vi "Get Named Range Values (Boolean).vi"(8 "error in":errorcluster, 9 "Sheet Name":string, 10 "Named Range Identifier":string, 11 "SpreadsheetDoc in":refnum<k24>) -> (0 "error out":errorcluster, 2 "Cells":bool[][](array[boolean]), 3 "SpreadsheetDoc out":refnum<k24>)   [LabVIEW 2019, in "Open Xml.lvlib"]
uses:
  Open Xml.lvlib
  D:/git/Open-Xml-LabVIEW/Source/DocumentFormat.OpenXml.dll
  DocumentFormat.OpenXml.dll
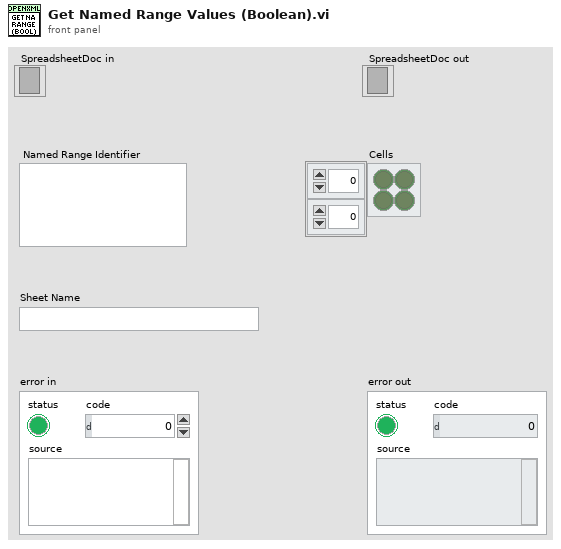
[diagram p1: front panel]
types:
  T1 = typedef "Open Xml.lvlib/Cell DataType.ctl" = enum16{"Void", "Boolean", "Number", "Error", "SharedString", "String", "InlineString", "Date"}
  T2 = cluster{"Number":dbl, "String":string, "Boolean":bool, "Time Stamp":timestamp, "Error":errorcluster}[][]
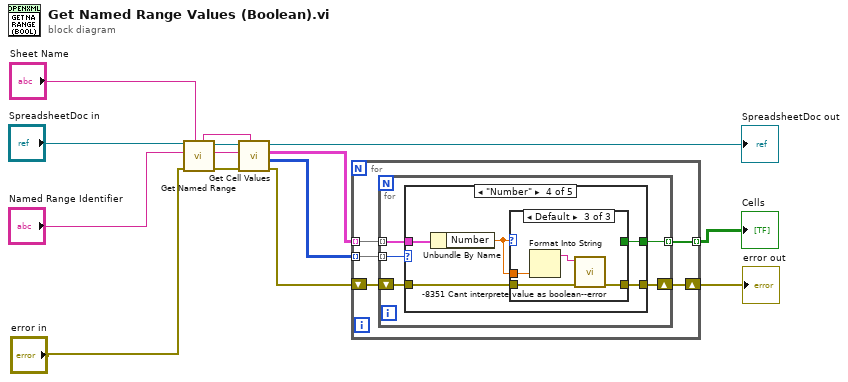
[diagram p0: block diagram]
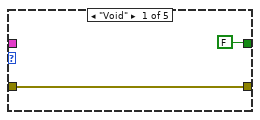
[diagram p2: hidden frame]
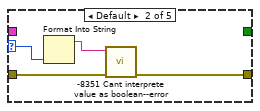
[diagram p3: hidden frame]
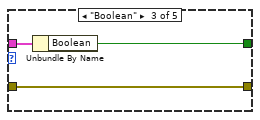
[diagram p4: hidden frame]
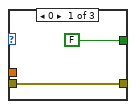
[diagram p5: hidden frame]
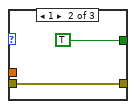
[diagram p6: hidden frame]
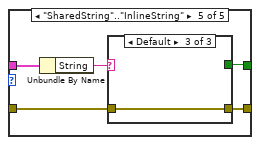
[diagram p7: hidden frame]
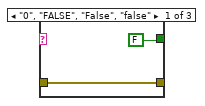
[diagram p8: hidden frame]
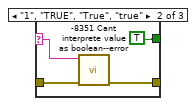
[diagram p9: hidden frame]
diagram:
  n1 = call "Get Named Range.vi"("Sheet Name"="Sheet Name", "error in"="error in", "Range Identifier"="Named Range Identifier", "SpreadsheetDoc in"="SpreadsheetDoc in") -> ("error out"=w11:errorcluster, "Range"=w8:string, "SpreadsheetDoc out"=w10:refnum<k24>, "Sheet Name"=w9:string)  [unwired: 4 in]
  n2 = call "Get Cell Values.vi"("Sheet Name"=w9, "error in"=w11, "Cell Addresses"=w8, "SpreadsheetDoc in"=w10) -> ("error out"=w3:errorcluster, "Types"=w5:T1[][], "Cell Values"=w7:T2, "SpreadsheetDoc out"=→"SpreadsheetDoc out":refnum<k24>)  [unwired: 4 in]
  n3 = for {
    tunnel: w7 -> [w19] mode=indexing
    tunnel: w5 -> [w18] mode=indexing
    tunnel: [w17] -> w1 mode=indexing
    shift-right: [w15] -> w2
    shift-left: w3 -> [w16]
    n4 = for {
      tunnel: w19 -> [w23] mode=indexing
      tunnel: w18 -> [w24] mode=indexing
      tunnel: [w20] -> w17 mode=indexing
      shift-right: [w21] -> w15
      shift-left: w16 -> [w22]
      n5 = case shown="\"Number\"" w24 {
        selector: w24 -> [_ w28 _ _ _]
        tunnel: w23 -> [_ _ w33 w38 w51]
        tunnel: [FALSE _ w32 w37 w49] -> w20
        tunnel: w22 -> [w25 w30 w31 w36 w48]
        tunnel: [w25 w29 w31 w35 w47] -> w21
        frame "Void" {
        }
        frame Default {
          n6 = Format Into String(w28) -> (resulting string=w27:string)  [unwired: 3 in, 1 out]
          n7 = call "-8351 Cant interprete value as boolean--error.vi"("error in"=w30, "Argument"=w27) -> ("error out"=w29:errorcluster)  [unwired: 8 in, 1 out]
        }
        frame "Boolean" {
          n8 = Unbundle By Name(w33) -> ("Boolean"=w32:bool)
        }
        frame "Number" {
          n9 = Unbundle By Name(w38) -> ("Number"=w34:dbl)
          n10 = case shown="Default" w34 {
            tunnel: [FALSE TRUE _] -> w37
            tunnel: w36 -> [w39 w41 w45]
            tunnel: [w39 w41 w46] -> w35
            tunnel: w34 -> [_ _ w44]
            frame 0 {
            }
            frame 1 {
            }
            frame Default {
              n11 = Format Into String(w44) -> (resulting string=w43:string)  [unwired: 3 in, 1 out]
              n12 = call "-8351 Cant interprete value as boolean--error.vi"("error in"=w45, "Argument"=w43) -> ("error out"=w46:errorcluster)  [unwired: 8 in, 1 out]
            }
          }
        }
        frame "SharedString".."InlineString" {
          n13 = Unbundle By Name(w51) -> ("String"=w50:string)
          n14 = case shown="Default" w50 {
            selector: w50 -> [_ w54 _]
            tunnel: [FALSE TRUE _] -> w49
            tunnel: w48 -> [w52 w56 w58]
            tunnel: [w52 w55 w58] -> w47
            frame "0", "FALSE", "False", "false" {
            }
            frame "1", "TRUE", "True", "true" {
              n15 = call "-8351 Cant interprete value as boolean--error.vi"("error in"=w56, "Argument"=w54) -> ("error out"=w55:errorcluster)  [unwired: 8 in, 1 out]
            }
            frame Default {
            }
          }
        }
      }
    }
  }
  "Cells" <- w1
  "error out" <- w2
